vi "readLogElevationAngleChecks.vi"(8 "error in (no error)":errorcluster, 10 "Parser":refnum<class "U8ArrayParserAutoIndexing.lvclass">, 11 "M1M3SAL in":refnum<class "M1M3SAL.lvclass">) -> (0 "error out":errorcluster, 2 "EventElevationAngleChecks":variant, 3 "M1M3SAL out":refnum<class "M1M3SAL.lvclass">)   [LabVIEW 2016, in "M1M3SupportCommunicator.lvlib" / "M1M3SAL.lvclass"]
uses:
  M1M3SAL.lvclass
  Common_RT_Utilities/U8ArrayParserAutoIndexing/U8ArrayParserAutoIndexing.lvclass
  DataTypes/Topics/EventElevationAngleChecks.ctl
  DataTypes/Topics/Parts/Timestamp.ctl
  DataTypes/Topics/M1M3SupportTopics.lvlib
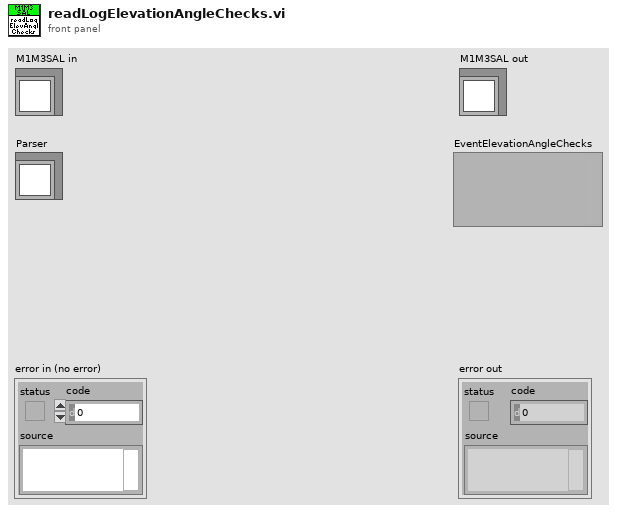
[diagram p1: front panel]
types:
  T1 = typedef "M1M3SupportTopics.lvlib/EventElevationAngleChecks.ctl" = cluster{"Timestamp":T2, "MatchesTMA":bool, "MatchesInclinometer":bool, "MatchesMeasured":bool}
  T2 = typedef "M1M3SupportTopics.lvlib/Timestamp.ctl" = dbl
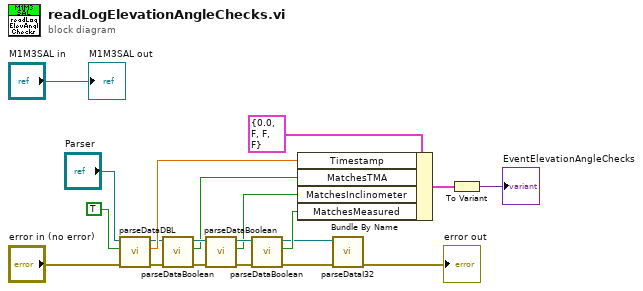
[diagram p0: block diagram]
diagram:
  n1 = call "parseDataDBL.vi"("error in (no error)"="error in (no error)", "OverrideSwapBytes"=TRUE, "U8ArrayParserAutoIndexing in"="Parser") -> ("error out"=w6:errorcluster, "Data"=w13:dbl, "U8ArrayParserAutoIndexing out"=w7:refnum<class "U8ArrayParserAutoIndexing.lvclass">)  [unwired: 6 in]
  n2 = call "parseDataBoolean.vi"("error in (no error)"=w6, "U8ArrayParserAutoIndexing in"=w7) -> ("error out"=w11:errorcluster, "Data"=w5:bool, "U8ArrayParserAutoIndexing out"=w10:refnum<class "U8ArrayParserAutoIndexing.lvclass">)  [unwired: 7 in]
  n3 = call "parseDataBoolean.vi"("error in (no error)"=w11, "U8ArrayParserAutoIndexing in"=w10) -> ("error out"=w9:errorcluster, "Data"=w4:bool, "U8ArrayParserAutoIndexing out"=w8:refnum<class "U8ArrayParserAutoIndexing.lvclass">)  [unwired: 7 in]
  n4 = call "parseDataBoolean.vi"("error in (no error)"=w9, "U8ArrayParserAutoIndexing in"=w8) -> ("error out"=w2:errorcluster, "Data"=w3:bool, "U8ArrayParserAutoIndexing out"=w1:refnum<class "U8ArrayParserAutoIndexing.lvclass">)  [unwired: 7 in]
  n5 = Bundle By Name(cluster=T1 {"Timestamp"=0.0, "MatchesTMA"=FALSE, "MatchesInclinometer"=FALSE, "MatchesMeasured"=FALSE} ("EventElevationAngleChecks"), "Timestamp"=w13, "MatchesTMA"=w5, "MatchesInclinometer"=w4, "MatchesMeasured"=w3) -> (w19:T1)
  n6 = call "parseDataI32.vi"("error in (no error)"=w2, "U8ArrayParserAutoIndexing in"=w1) -> ("error out"=→"error out":errorcluster)  [unwired: 7 in, 2 out]
  n7 = To Variant(anything=w19) -> (Variant=→"EventElevationAngleChecks":variant)
  "M1M3SAL out" <- "M1M3SAL in"
